vi "Read Inventario.vi"(8 "error in":errorcluster) -> (0 "error out":errorcluster, 3 "Inventario":T1)   [LabVIEW 2024, in "ProductControl.lvlib"]
uses:
  ProductControl.lvlib
  <vilib>/Utility/file.llb/Application Directory.vi
  <vilib>/Utility/config.llb/Read Key (U32).vi
  <vilib>/Utility/config.llb/Read Key (Double).vi
  <vilib>/Utility/config.llb/NI_LVConfig.lvlib
  Products--array.ctl
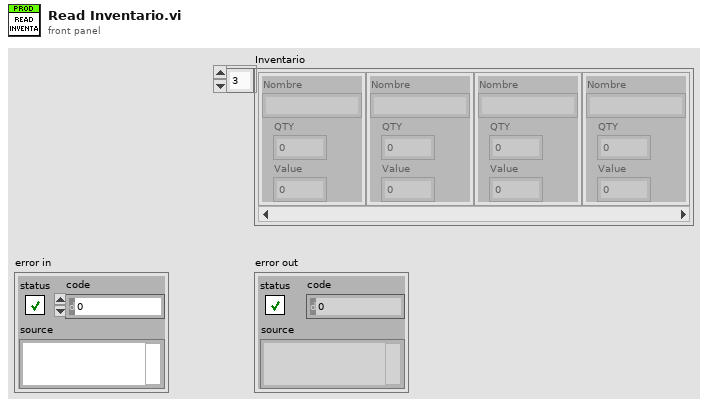
[diagram p1: front panel]
types:
  T1 = typedef "ProductControl.lvlib/Products--array.ctl" = cluster{"Nombre":string, "QTY":u32, "Value":dbl}[]
  T2 = typedef "NI_LVConfig.lvlib/Config Data RefNum.ctl" = refnum<k1>
  T3 = cluster{"String":string, "value":u32, "value":dbl}
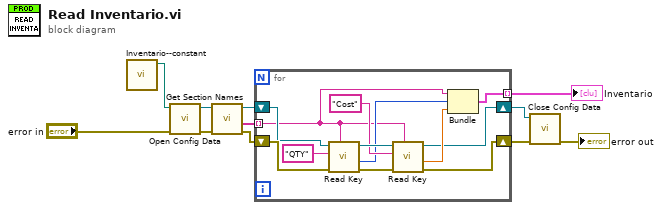
[diagram p0: block diagram]
diagram:
  n1 = call "Inventario--constant.vi"() -> ("Path"=w6:path)  [unwired: 11 in]
  n2 = call <vilib>:"Open Config Data.vi"("error in (no error)"="error in", "configuration file path"=w6) -> ("error out"=w11:errorcluster, "refnum"=w5:T2)  [unwired: 7 in, 1 out]
  n3 = call <vilib>:"Get Section Names.vi"("error in (no error)"=w11, "refnum"=w5) -> ("error out"=w10:errorcluster, "section names"=w4:string[], "refnum out"=w3:T2)  [unwired: 7 in]
  n4 = for {
    tunnel: w4 -> [w12] mode=indexing
    shift-right: [w14] -> w2
    shift-left: w3 -> [w20]
    shift-right: [w21] -> w9
    shift-left: w10 -> [w23]
    tunnel: [w13] -> w1 mode=indexing
    n5 = call-poly <vilib>:"Read Key.vi"("section"=w12, "error in (no error)"=w23, "key"="QTY", "refnum"=w20) -> ("error out"=w22:errorcluster, "value"=w16:u32, "refnum out"=w18:T2)  [unwired: 4 in, 1 out]
    n6 = call-poly <vilib>:"Read Key.vi"("section"=w12, "error in (no error)"=w22, "key"="Cost", "refnum"=w18) -> ("error out"=w21:errorcluster, "value"=w15:dbl, "refnum out"=w14:T2)  [unwired: 4 in, 1 out]
    n7 = Bundle("String"=w12, "value"=w16, "value"=w15) -> (w13:T3)  [unwired: 1 in]
  }
  "Inventario" <- w1
  n8 = call <vilib>:"Close Config Data.vi"("error in (no error)"=w9, "refnum"=w2) -> ("error out"=→"error out":errorcluster)  [unwired: 8 in, 1 out]
